vi "rad_RePackNestedImage.vi"(8 "error in (no error)":errorcluster, 10 "Unzipped files":path[](array[path]), 11 "target":path) -> (0 "error out":errorcluster, 3 "target out":path)   [LabVIEW 2023]
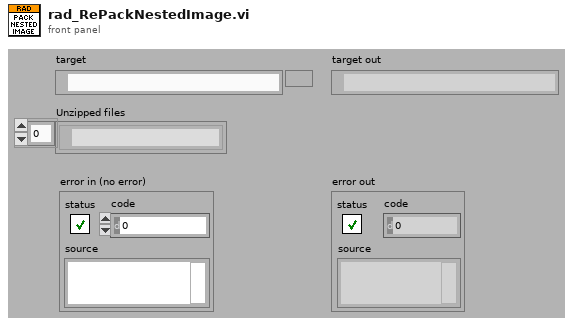
[diagram p1: front panel]
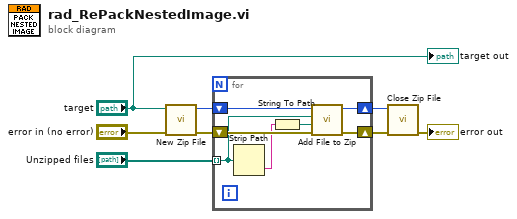
[diagram p0: block diagram]
diagram:
  n1 = call <vilib>:"New Zip File.vi"("error in (no error)"="error in (no error)", "target"="target") -> ("error out"=w6:errorcluster, "zip file out"=w5:i64)  [unwired: 3 in, 1 out]
  n2 = for {
    tunnel: "Unzipped files" -> [w13] mode=indexing
    shift-right: [w10] -> w3
    shift-left: w6 -> [w14]
    shift-right: [w9] -> w4
    shift-left: w5 -> [w15]
    n3 = Strip Path(path=w13) -> (name=w12:string)  [unwired: 1 out]
    n4 = String To Path(string=w12) -> (path=w11:path)
    n5 = call <vilib>:"Add File to Zip.vi"("error in (no error)"=w14, "destination path in zip"=w11, "source file path"=w13, "zip file in"=w15) -> ("error out"=w10:errorcluster, "zip file out"=w9:i64)  [unwired: 6 in]
  }
  n6 = call <vilib>:"Close Zip File.vi"("error in (no error)"=w3, "zip file in"=w4) -> ("error out"=→"error out":errorcluster)  [unwired: 5 in]
  "target out" <- "target"
